vi "Create Data Channel Element.vi"(6 "Data Channel Parameters":T3, 7 "Settings":T1, 8 "Error In":errorcluster, 10 "Name":string, 11 "Refnum In":T8 format="%.0x") -> (0 "Error Out":errorcluster, 2 "Channel Refnum":T8 format="%.0x", 3 "Refnum Out":T8 format="%.0x")   [LabVIEW 2018, in "Instrument Addon Scripting API.lvlib"]
uses:
  Instrument Addon Scripting API.lvlib
  <vilib>/NI Veristand/Custom Device API/Custom Device Item Ref.ctl
  Addon/Addon Shared/Types/Data Parameters.ctl
  Addon/Addon Shared/Types/Protocol Data Type.ctl
  Addon/Addon Shared/Types/Data Channel Type.ctl
  Addon/Addon Shared/Types/Type Cast Type.ctl
  Addon/Addon Shared/Types/Endian.ctl
  <vilib>/NI Veristand/Custom Device API/Custom Device Channel.ctl
  <vilib>/NI Veristand/Custom Device API/Custom Device Channel Type.ctl
  Addon/Addon Shared/Types/FG Control.ctl
  Addon/Addon Shared/SubVIs/Constants.vi
  <vilib>/NI Veristand/Custom Device API/Custom Device API.lvlib
  Addon/Addon Shared/Instrument Addon Shared.lvlib
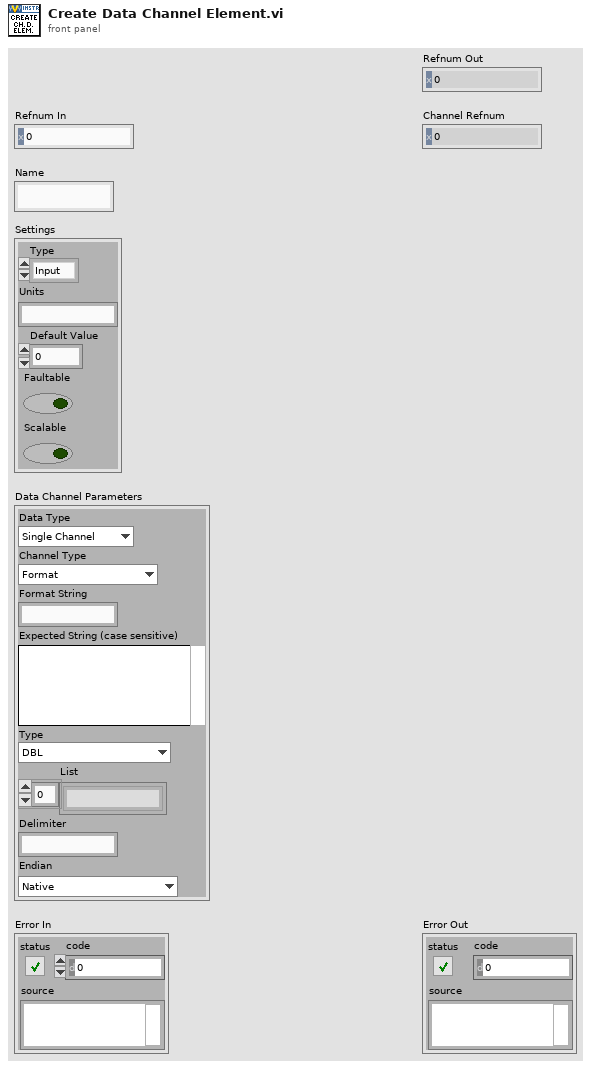
[diagram p1: front panel]
types:
  T1 = typedef "Custom Device API.lvlib/Custom Device Channel.ctl" = cluster{"Type":T2, "Units":string, "Default Value":dbl, "Faultable":bool, "Scalable":bool}
  T2 = typedef "Custom Device API.lvlib/Custom Device Channel Type.ctl" = enum16{"Input", "Output"}
  T3 = typedef "Instrument Addon Shared.lvlib/Data Parameters.ctl" = cluster{"Data Type":T4, "Channel Type":T5, "Format String":string, "Expected String":string, "Type":T6, "List":string[], "Delimiter":string, "Endian":T7}
  T4 = typedef "Instrument Addon Shared.lvlib/Protocol Data Type.ctl" = enum16{"Single Channel", "Array"}
  T5 = typedef "Instrument Addon Shared.lvlib/Data Channel Type.ctl" = enum16{"Format", "Comparison", "Type Cast", "Enumerated List"}
  T6 = typedef "Instrument Addon Shared.lvlib/Type Cast Type.ctl" = enum16{"DBL", "SGL", "U64", "U32", "U16", "U8", "I64", "I32", "I16", "I8"}
  T7 = typedef "Instrument Addon Shared.lvlib/Endian.ctl" = enum16{"Native", "Little", "Big"}
  T8 = typedef "Custom Device API.lvlib/Custom Device Item Ref.ctl" = u64
  T9 = typedef "Instrument Addon Shared.lvlib/FG Control.ctl" = enum16{"Get", "Set"}
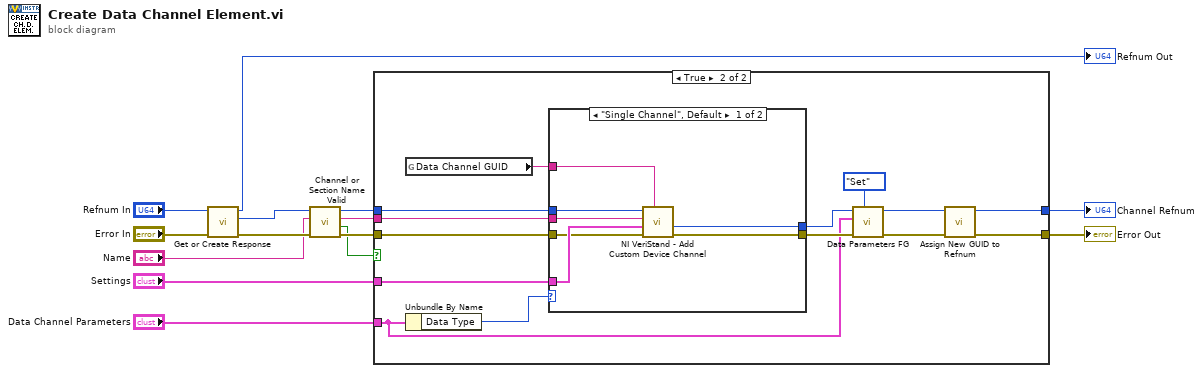
[diagram p0: block diagram]
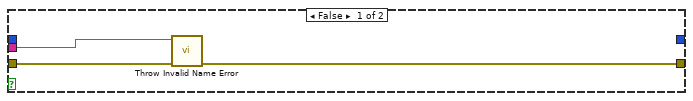
[diagram p2: hidden frame]
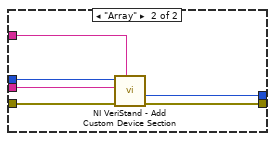
[diagram p3: hidden frame]
diagram:
  n1 = call "Get or Create Response.vi"("Error In"="Error In", "Message Refnum In in"="Refnum In") -> ("Error Out"=w7:errorcluster, "Response Refnum"=w8:T8, "Message Refnum Out"=→"Refnum Out":T8)  [unwired: 7 in]
  n2 = call "Channel or Section Name Valid.vi"("error in (no error)"=w7, "Name In"="Name", "Refnum In"=w8) -> ("error out"=w5:errorcluster, "Name Valid?"=w2:bool, "Name Out"=w3:string, "Refnum Out"=w4:T8)  [unwired: 5 in]
  n3 = case shown="True" w2 {
    tunnel: [_ w19] -> w14
    tunnel: "Settings" -> [_ w31]
    tunnel: [w15 w18] -> w12
    tunnel: "Data Channel Parameters" -> [_ w24]
    tunnel: w5 -> [w17 w26]
    tunnel: w4 -> [_ w25]
    tunnel: w3 -> [w16 w23]
    frame False {
      n4 = call "Throw Invalid Name Error.vi"("error in (no error)"=w17, "Name"=w16) -> ("error out"=w15:errorcluster)  [unwired: 9 in]
    }
    frame True {
      n5 = global read "Constants.vi" "Data Channel GUID"() -> (w22:string)
      n6 = Unbundle By Name(w24) -> ("Data Type"=w27:T4)
      n7 = case shown="\"Single Channel\", Default" w27 {
        tunnel: w23 -> [w38 w44]
        tunnel: w31 -> [w37 _]
        tunnel: [w36 w39] -> w29
        tunnel: [w35 w40] -> w28
        tunnel: w26 -> [w34 w42]
        tunnel: w25 -> [w33 w41]
        tunnel: w22 -> [w32 w43]
        frame "Single Channel", Default {
          n8 = call <vilib>:"NI VeriStand - Add Custom Device Channel.vi"("GUID (Default Channel)"=w32, "error in (no error)"=w34, "Channel"=w37, "Channel Name"=w38, "Parent Ref in"=w33) -> ("error out"=w35:errorcluster, "Channel Ref"=w36:T8)  [unwired: 3 in, 2 out]
        }
        frame "Array" {
          n9 = call <vilib>:"NI VeriStand - Add Custom Device Section.vi"("GUID (Default Section)"=w43, "error in (no error)"=w42, "Section Name"=w44, "Parent Ref in"=w41) -> ("error out"=w40:errorcluster, "Section Ptr"=w39:T8)  [unwired: 4 in, 2 out]
        }
      }
      n10 = call "Data Parameters FG.vi"("Action"=FG_Control."Set", "error in (no error)"=w28, "Data Parameters"=w24, "Item Ref in"=w29) -> ("error out"=w21:errorcluster, "Item Ref out"=w20:T8)  [unwired: 5 in, 1 out]
      n11 = call "Assign New GUID to Refnum.vi"("error in (no error)"=w21, "Item Ref in"=w20) -> ("error out"=w18:errorcluster, "Item Ref out"=w19:T8)  [unwired: 8 in]
    }
  }
  "Channel Refnum" <- w14
  "Error Out" <- w12
